vi "Config has been set.vi"(8 "error in":errorcluster, 10 "Sim Signal Config":T1={"offset"=0.0, "square wave duty cycle (%)"=50.0, "signal type"=enum."Sine Wave", "phase"=0.0, "amplitude"=1.0, "frequency"=10.0, "sampling info"={"Fs"=1000.0, "#s"=1000.0}} {"sampling info"."Fs" format="%.2p"; "frequency" scale=0.0..10.0; "amplitude" scale=0.0..10.0; "phase" format="%.2p"; "square wave duty cycle (%)" format="%0.2f"; "offset" scale=0.0..10.0}) -> (0 "error out":errorcluster)   [LabVIEW 2020, in "Config.lvlib"]
doc: "Config has been set\n_____\nCreated using Delacor QMH Event Scripter 6.0.0.121."
uses:
  Config.lvlib
  sim signal -- cluster.ctl
  Config has been set Argument--cluster.ctl
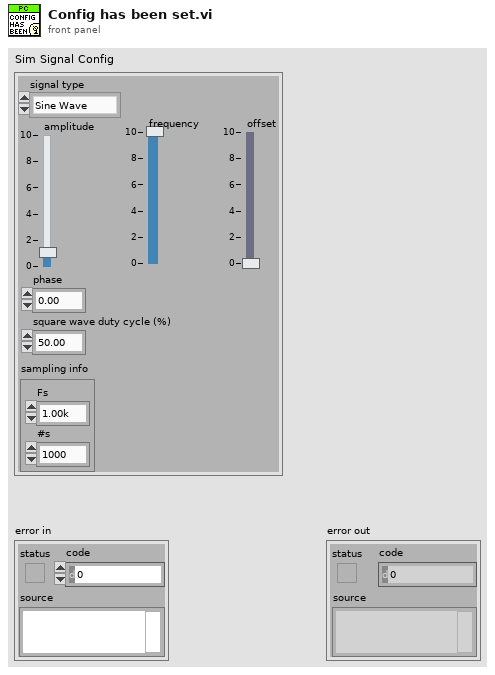
[diagram p1: front panel]
types:
  T1 = typedef "Config.lvlib/sim signal -- cluster.ctl" = cluster{"offset":dbl, "square wave duty cycle (%)":dbl, "signal type":enum16{"Sine Wave", "Triangle Wave", "Square Wave", "Sawtooth Wave"}, "phase":dbl, "amplitude":dbl, "frequency":dbl, "sampling info":cluster{"Fs":dbl, "#s":dbl}}
  T2 = typedef "Config.lvlib/Config has been set Argument--cluster.ctl" = cluster{"Sim Signal Config":T1}
  T3 = typedef "Config.lvlib/Broadcast Events--cluster.ctl" = cluster{"Module Did Init":refnum<user-event>, "Status Updated":refnum<user-event>, "Error Reported":refnum<user-event>, "Module Did Stop":refnum<user-event>, "Update Module Execution Status":refnum<user-event>, "Config has been set":refnum<user-event>}
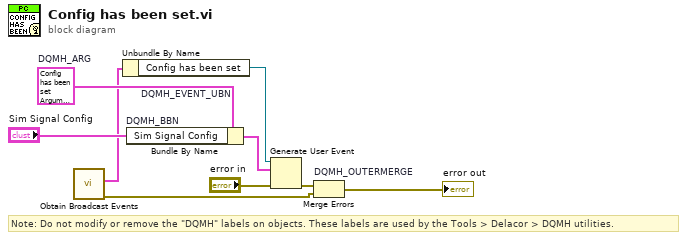
[diagram p0: block diagram]
diagram:
  w4 = T2 {"Sim Signal Config"={"offset"=0.0, "square wave duty cycle (%)"=50.0, "signal type"=enum."Sine Wave", "phase"=0.0, "amplitude"=1.0, "frequency"=10.0, "sampling info"={"Fs"=1000.0, "#s"=1000.0}}}  # DQMH_ARG
  # "Note: Do not modify or remove the \"DQMH\" labels on objects. These labels are used by the Tools > Delacor > DQMH utilities."
  n1 = call "Obtain Broadcast Events.vi"() -> ("error out"=w2:errorcluster, "Config Broadcast Events"=w1:T3)  [unwired: 10 in]
  n2 = Unbundle By Name "DQMH_EVENT_UBN"(w1) -> ("Config has been set"=w6:refnum<user-event>)
  n3 = Bundle By Name "DQMH_BBN"(cluster=w4, "Sim Signal Config"="Sim Signal Config") -> (w7:T2)
  n4 = Generate User Event(user event=w6, event data cluster=w7, error in="error in") -> (error out=w5:errorcluster)  [unwired: 1 in, 1 out]
  n5 = Merge Errors "DQMH_OUTERMERGE"(w5, w2) -> (→"error out":errorcluster)
